vi "CVT2LoadDeprecatedTags.vi"() -> (3 "Unit Test Framework Results":T1)   [LabVIEW 2013, in "UnitTests.lvlib"]
doc: "Use this template to create a user-defined test VI. Define your test requirements and wire the results to the <b>Result (Test)</b> control. Do not modify the <b>Unit Test Framework Results</b> indicator."
uses:
  UnitTests.lvlib
  <vilib>/utf/common/utf_test_result_troll.ctl
  <vilib>/utf/common/utf_test_result.ctl
  <vilib>/utf/common/utf_test_result_failure.ctl
  <vilib>/utf/common/utf_test_comparison_operators.ctl
  <vilib>/utf/common/utf_vi_tag.ctl
  <vilib>/NI/Current Value Table/DataTypes/I32_Read.vi
  <vilib>/NI/Current Value Table/Type to Enum.vi
  <vilib>/NI/Current Value Table/DataTypes/I32_Type To Enum.vi
  <vilib>/NI/Current Value Table/Compatibility/TagConverter.vi
  <vilib>/NI/Current Value Table/Create Tags.vi
  <vilib>/NI/Current Value Table/FGVs/CVT Globals.vi
  <vilib>/NI/Current Value Table/FGVs/Tag Memory.vi
  <vilib>/NI/Current Value Table/Memory Block.vi
  <vilib>/NI/Current Value Table/DataTypes/I32_Memory Block.vi
  <vilib>/utf/NI_UnitTestFramework.lvlib
  <vilib>/NI/Current Value Table/Current Value Table.lvlib
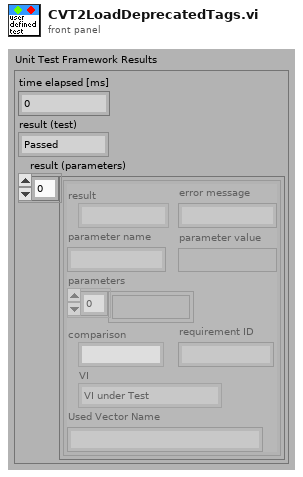
[diagram p1: front panel]
types:
  T1 = typedef "NI_UnitTestFramework.lvlib/utf_test_result_troll.ctl" = cluster{"time elapsed [ms]":u32, "result (test)":T2, "result (parameters)":T3[]}
  T2 = typedef "NI_UnitTestFramework.lvlib/utf_test_result.ctl" = enum16{"Passed", "Failed", "Error", "Skipped", "Not Processed"}
  T3 = typedef "NI_UnitTestFramework.lvlib/utf_test_result_failure.ctl" = cluster{"result":T2, "error message":string, "parameter name":string, "parameter value":variant, "parameters":variant[], "comparison":T4, "requirement ID":string, "VI":T5, "Used Vector Name":string}
  T4 = typedef "NI_UnitTestFramework.lvlib/utf_test_comparison_operators.ctl" = enum16{"=", "!=", ">", ">=", "<", "<=", "range", "symmetric tolerance", "asymmetric tolerance", "string contains", "string not contain", "array size", "string length", "array range", "by element", "array range (limit array)", "user-defined", "array contains", "array not contain", "vector length", "= (elm)", "!= (elm)", "= (case insensitive)", "!= (case insensitive)"}
  T5 = typedef "NI_UnitTestFramework.lvlib/utf_vi_tag.ctl" = enum16{"Setup VI", "VI under Test", "Teardown VI"}
  T6 = typedef "cvt_Tag Configuration.ctl" = cluster{"Name":string, "Data Type":T7, "Array":bool, "Size":u32, "Default":string, "Enum":string[], "Description":string}
  T7 = typedef "cvt_Data Types.ctl" = enum16{"Bool", "U8", "I32", "Double", "String", "Enum"}
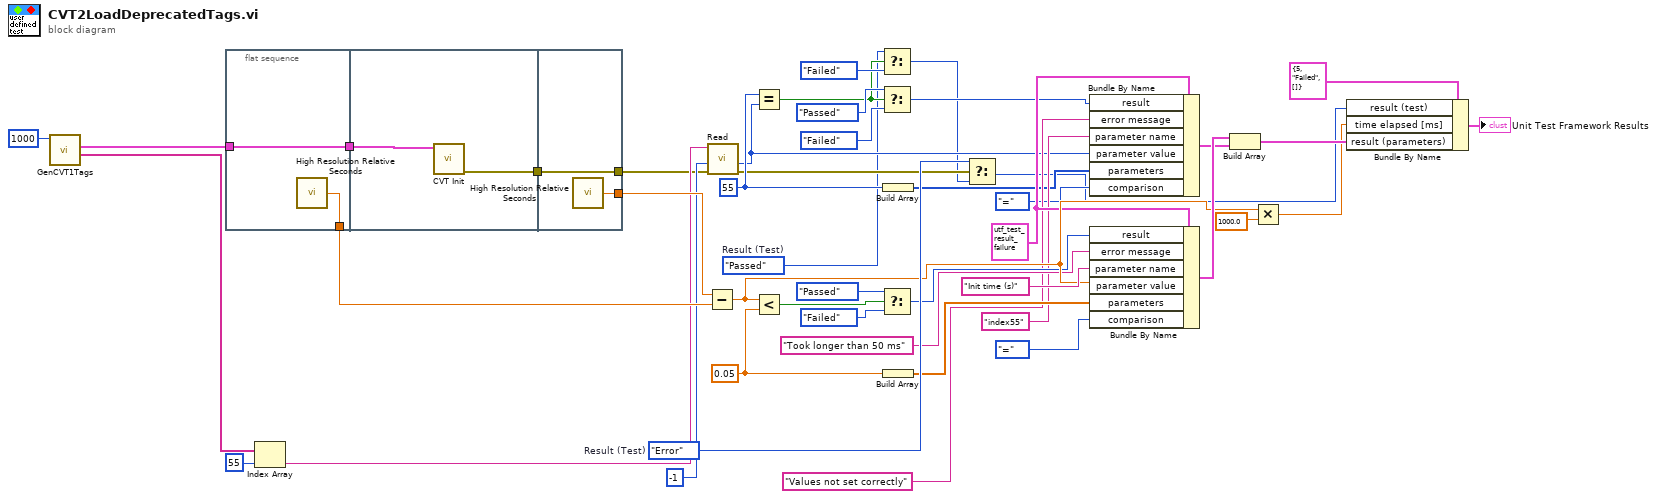
[diagram p0: block diagram]
diagram:
  w17 = 55 ("Index")
  w30 = 0.05 ("y")
  w25 = T3 {"result"=enum."Passed", "error message"="", "parameter name"="", "parameter value"=variant, "parameters"=[], "comparison"=enum."=", "requirement ID"="", "VI"=enum."Setup VI", "Used Vector Name"=""} ("Unit Test Framework - result (parameters)")
  w41 = utf_test_result."Error"  # Result (Test)
  w10 = utf_test_result."Passed"  # Result (Test)
  n1 = call "GenCVT1Tags.vi"("Number of Tags in"=1000) -> ("Names"=w6:string[], "Tags"=w1:T6[])  [unwired: 8 in, 1 out]
  n2 = flat-sequence {
    tunnel: [w47] -> w43
    tunnel: [w46] -> w2
    tunnel: w1 -> [w46]
    tunnel: [w49] -> w3
    tunnel: w2 -> [w48]
    tunnel: [w51] -> w44
    tunnel: [w50] -> w4
    tunnel: w3 -> [w50]
    frame #0 {
      n3 = call <vilib>:"High Resolution Relative Seconds.vi"() -> ("relative seconds"=w47:dbl)
    }
    frame #1 {
      n4 = call <vilib>:"CVT Init.vi"("Tag List"=w48) -> ("error out"=w49:errorcluster)  [unwired: 10 in]
    }
    frame #2 {
      n5 = call <vilib>:"High Resolution Relative Seconds.vi"() -> ("relative seconds"=w51:dbl)
    }
  }
  n6 = Index Array(array=w6, index=55) -> (element=w5:string)
  n7 = Subtract(x=w44, y=w43) -> (x-y=w36:dbl)
  n8 = call-poly <vilib>:"Read.vi"("error in (no error)"=w4, "Default"=-1, "Tag Name"=w5) -> ("error out"=w11:errorcluster, "Value"=w12:i32)  [unwired: 7 in]
  n9 = Equal?(x=w17, y=w12) -> (x = y?=w21:bool)
  n10 = Less?(x=w36, y=w30) -> (x < y?=w29:bool)
  n11 = Select(t=w10, s=w21, f=utf_test_result."Failed") -> (s? t:f=w8:T2)
  n12 = Select(t=utf_test_result."Passed" ("result"), s=w21, f=utf_test_result."Failed" ("result")) -> (s? t:f=w22:T2)
  n13 = Select(t=utf_test_result."Passed" ("result"), s=w29, f=utf_test_result."Failed" ("result")) -> (s? t:f=w35:T2)
  n14 = Build Array(w17) -> (w18:i32[])
  n15 = Build Array(w30) -> (w31:dbl[])
  n16 = Select(t=w41, s=w11, f=w8) -> (s? t:f=w9:T2)
  n17 = Bundle By Name(cluster=w25, "result"=w22, "error message"="Values not set correctly", "parameter name"="index55", "parameter value"=w12, "parameters"=w18, "comparison"=utf_test_comparison_operators."=") -> (w26:T3)
  n18 = Bundle By Name(cluster=w25, "result"=w35, "error message"="Took longer than 50 ms", "parameter name"="Init time (s)", "parameter value"=w36, "parameters"=w31, "comparison"=utf_test_comparison_operators."=") -> (w40:T3)
  n19 = Build Array(w40, w26) -> (w39:T3[])
  n20 = Multiply(x=w36, y=1000.0) -> (x*y=w37:dbl)
  n21 = Bundle By Name(cluster=T1 {"time elapsed [ms]"=5, "result (test)"=enum."Failed", "result (parameters)"=[]} ("Unit Test Framework - Result"), "result (test)"=w9, "time elapsed [ms]"=w37, "result (parameters)"=w39) -> (→"Unit Test Framework Results":T1)
